vi "Keysight 34401A Check Range.vi"(3 "value":dbl) -> (1 "out of range?":bool)   [LabVIEW 2020, in "Keysight 34401A DMM Measurement.lvlib"]
uses:
  Keysight 34401A DMM Measurement.lvlib
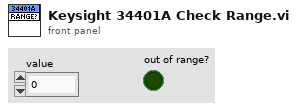
[diagram p1: front panel]
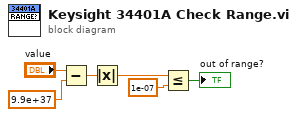
[diagram p0: block diagram]
diagram:
  n1 = Subtract(x="value", y=9.9e+37) -> (x-y=w4:dbl)
  n2 = Absolute Value(x=w4) -> (abs(x)=w3:dbl)
  n3 = Less Or Equal?(x=w3, y=1e-07) -> (x <= y?=→"out of range?":bool)
